vi "NET EnableWinograd.vi"(8 "error in (no error)":errorcluster, 10 "UseWinograd":bool=TRUE, 11 "NET in":refnum<class "NET.lvclass">) -> (0 "error out":errorcluster, 3 "NET out":refnum<class "NET.lvclass">)   [LabVIEW 2020, in "OpenLvVision_OpenCv.lvlib" / "NET.lvclass"]
doc: "Enables or disables the Winograd compute branch. The Winograd compute branch can speed up 3x3 Convolution at a small loss of accuracy."
uses:
  NET.lvclass
  C:/Users/lukas/Downloads/OpenLvVision_OpenCv/SourceCode/LabView/OpenLvVision_OpenCv/_LvHelpers/EdvrObject/EdvrObject.lvclass
  _LvHelpers/EdvrObject/EdvrObject.lvclass/EdvrObject.ctl
  OpenLvVision_OpenCv.lvlib
  _LvHelpers/EdvrObject/EdvrObject.lvclass
  Dlls/OlvOpenCvWrapper.dll
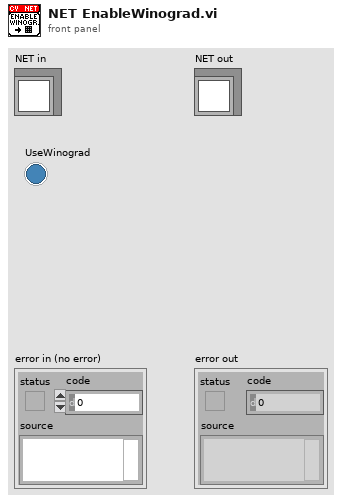
[diagram p1: front panel]
types:
  T1 = typedef "OpenLvVision_OpenCv.lvlib/EdvrObject.lvclass/Edvr.ctl" = refnum<data-value>
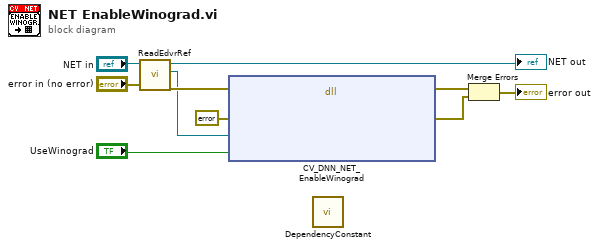
[diagram p0: block diagram]
diagram:
  n1 = call "ReadEdvrRef.vi"("error in (no error)"="error in (no error)", "EdvrObject in"="NET in") -> ("error out"=w6:errorcluster, "Edvr"=w5:T1, "EdvrObject out"=→"NET out":refnum<class "NET.lvclass">)  [unwired: 7 in]
  n2 = dll-call lib="C:/Users/lukas/Downloads/OpenLvVision_OpenCv/SourceCode/LabView/OpenLvVision_OpenCv/Dlls/OlvOpenCvWrapper.dll" fn="CV_DNN_NET_EnableWinograd"(error in=w6, "Error"=errorcluster {"status"=FALSE, "code"=0, "source"=""} ("error out"), "edvrRef"=w5, "useWinograd"="UseWinograd") -> (error out=w9:errorcluster, "Error"=w2:errorcluster)  [unwired: 5 in, 1 out]
  n3 = call "DependencyConstant.vi"() -> ()  [unwired: 12 in]
  n4 = Merge Errors(w9, w2) -> (→"error out":errorcluster)
